vi "Spectro-ScanB.vi"(4 "Wrapp in":i32, 5 "Spectrometer num":i32, 6 "Boxcar":dbl=1.0 min=1.0 max=1000.0 step=1.0, 7 "Average":dbl=1.0 min=1.0 max=1000.0 step=1.0, 8 "Integration (ms)":dbl=10.0 min=1.0 max=1000.0 step=1.0 format="%#_2f", 9 "Spectrometer Selection":u16=1) -> (0 "Ocean Optics Spectrometer Single Scan Program":T1(graph), 1 "Spectral PowerBD":dbl[](array[numeric]), 2 "Spectral Power":dbl[](array[numeric]) format="%.1e", 3 "Wavelength (nm)":dbl[](array[numeric]) format="%.1f")   [LabVIEW 2017]
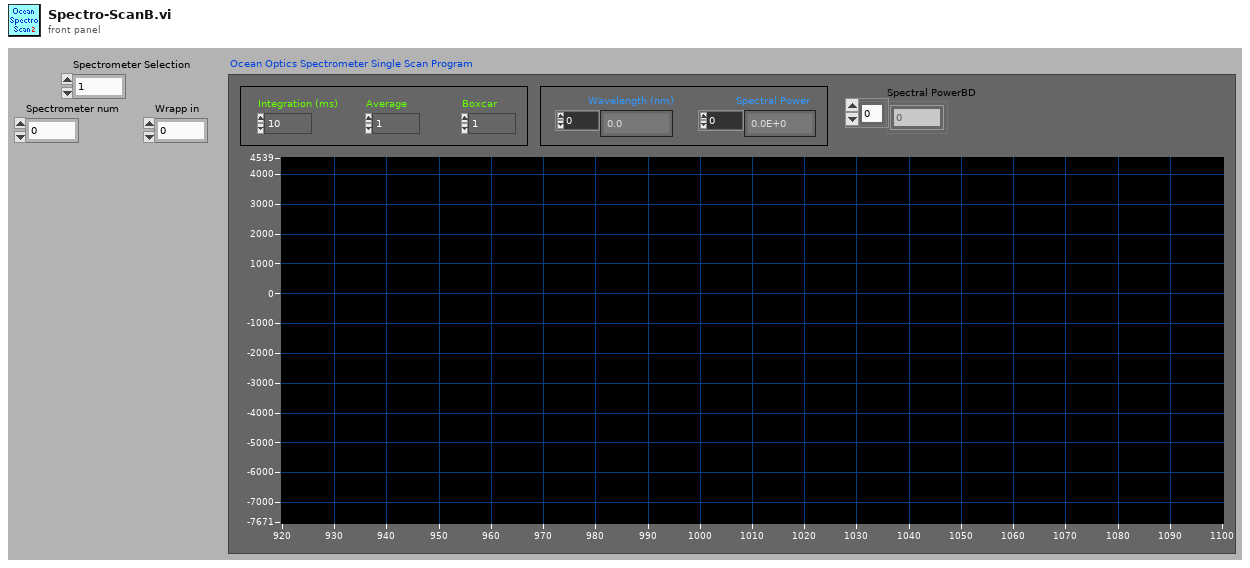
[diagram p1: front panel]
types:
  T1 = cluster{"WL Values":dbl[], "Spectrum Values":dbl[]}
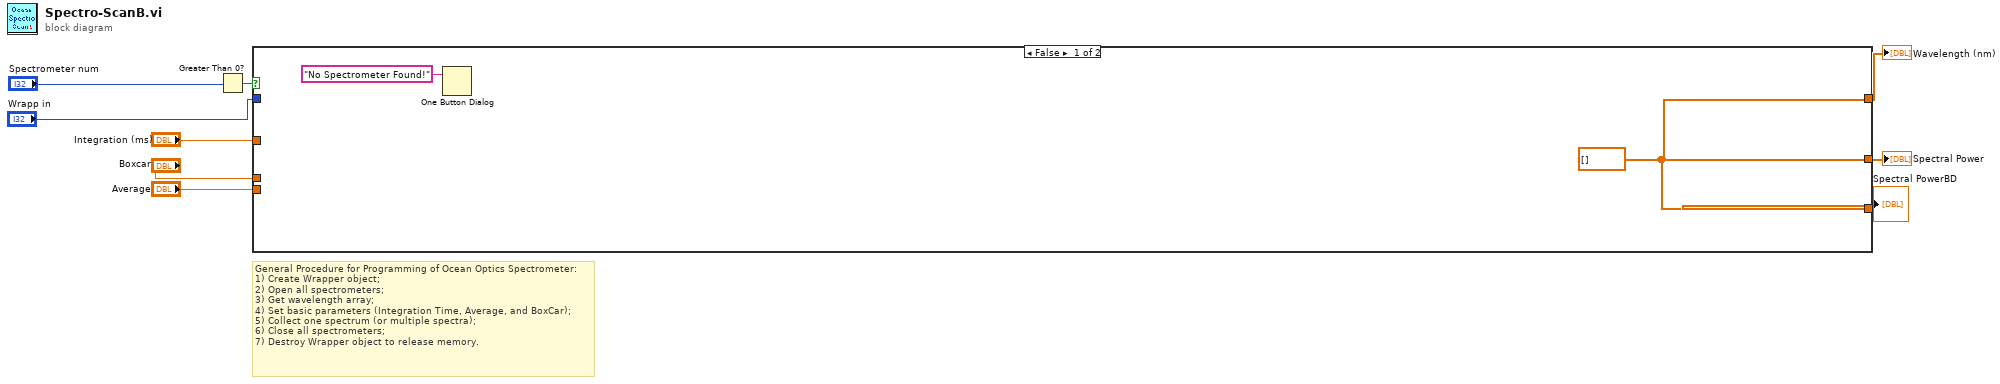
[diagram p0: block diagram]
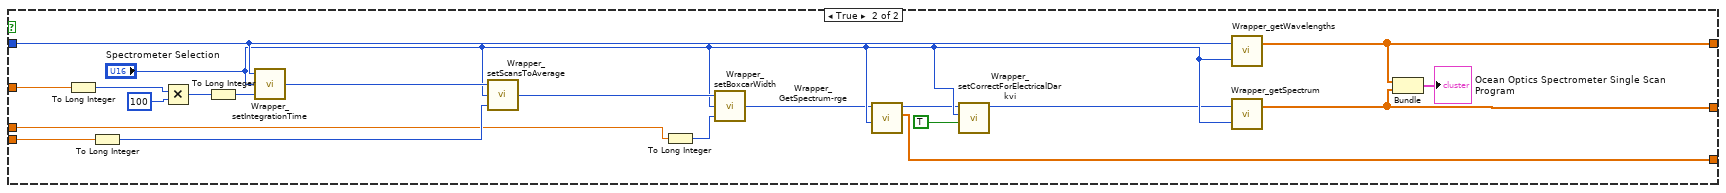
[diagram p2: hidden frame]
diagram:
  # "General Procedure for Programming of Ocean Optics Spectrometer:\n1) Create Wrapper object;\n2) Open all spectrometers;\n3) Get wavelength array;\n4) Set basic parameters (Integration Time, Average, and BoxCar);\n5) Collect one spectrum (or multiple spectra);\n6) Close all spectrometers;\n7) Destroy Wrapper object to release memory."
  n1 = Greater Than 0?(x="Spectrometer num") -> (x > 0?=w9:bool)
  n2 = case shown="False" w9 {
    tunnel: "Wrapp in" -> [_ w32]
    tunnel: [w10 w28] -> w8
    tunnel: [w10 w27] -> w7
    tunnel: [w10 w20] -> w6
    tunnel: "Integration (ms)" -> [_ w18]
    tunnel: "Average" -> [_ w16]
    tunnel: "Boxcar" -> [_ w13]
    frame False {
      w10 = dbl[] []
      n3 = One Button Dialog(message="No Spectrometer Found!") -> ()  [unwired: 1 in, 1 out]
    }
    frame True {
      n4 = To Long Integer(number=w18) -> (32bit integer=w17:i32)
      n5 = To Long Integer(number=w16) -> (32bit integer=w15:i32)
      n6 = Multiply(x=w17, y=100) -> (x*y=w26:i32)
      n7 = To Long Integer(number=w26) -> (32bit integer=w25:i32)
      n8 = call "Wrapper_setIntegrationTime.vi"("Integration Time"=w25, "Index"="Spectrometer Selection", "Wrapper In"=w32) -> ("Wrapper Out"=w30:u32)
      n9 = call "Wrapper_setScansToAverage.vi"("Average"=w15, "Index"="Spectrometer Selection", "Wrapper In"=w30) -> ("Wrapper Out"=w29:u32)
      n10 = To Long Integer(number=w13) -> (32bit integer=w14:i32)
      n11 = call "Wrapper_setBoxcarWidth.vi"("Boxcar Width"=w14, "Index"="Spectrometer Selection", "Wrapper In"=w29) -> ("Wrapper Out"=w22:u32)
      n12 = call "Wrapper_GetSpectrum-rge.vi"("Index"="Spectrometer Selection", "Wrapper"=w22) -> ("Spectrum Values"=w20:dbl[], "Wrapper out"=w21:u32)  [unwired: 7 in, 1 out]
      n13 = call "Wrapper_setCorrectForElectricalDarkvi.vi"("enableFlag"=TRUE, "Index in"="Spectrometer Selection", "Wrapper in"=w21) -> ("Wrapper out"=w19:u32)  [unwired: 7 in, 1 out]
      n14 = call "Wrapper_getWavelengths.vi"("Index"="Spectrometer Selection", "Wrapper"=w32) -> ("WL Values"=w28:dbl[])  [unwired: 1 out]
      n15 = call "Wrapper_getSpectrum.vi"("Index"="Spectrometer Selection", "Wrapper"=w19) -> ("Spectrum Values"=w27:dbl[])  [unwired: 1 out]
      n16 = Bundle("WL Values"=w28, "Spectrum Values"=w27) -> (→"Ocean Optics Spectrometer Single Scan Program":T1)  [unwired: 1 in]
    }
  }
  "Spectral Power" <- w7
  "Wavelength (nm)" <- w8
  "Spectral PowerBD" <- w6
